vi "GainsToString.vi"(11 "Gains":T2) -> (3 "Strings":string[](array[string]))   [LabVIEW 2017]
uses:
  <vilib>/Analysis/Matrix/Datatypes/RealMatrix.ctl
  <vilib>/Analysis/Matrix/NI_Matrix.lvlib
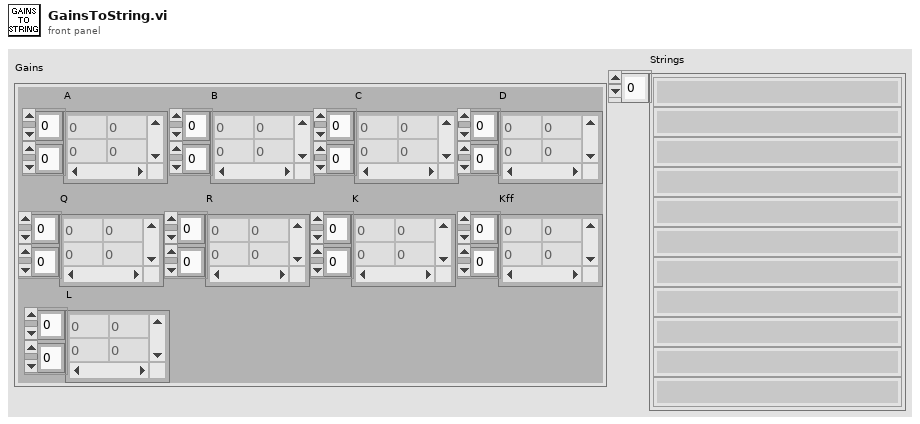
[diagram p1: front panel]
types:
  T1 = typedef "NI_Matrix.lvlib/RealMatrix.ctl" = dbl[][]
  T2 = cluster{"A":T1, "B":T1, "C":T1, "D":T1, "Q":T1, "R":T1, "K":T1, "Kff":T1, "L":T1}
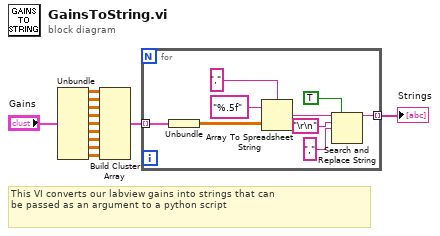
[diagram p0: block diagram]
diagram:
  # "This VI converts our labview gains into strings that can\nbe passed as an argument to a python script"
  n1 = Unbundle("Gains") -> ("A"=w1:T1, "B"=w11:T1, "C"=w10:T1, "D"=w9:T1, "Q"=w8:T1, "R"=w2:T1, "K"=w7:T1, "Kff"=w6:T1, "L"=w5:T1)
  n2 = Build Cluster Array(w1, w11, w10, w9, w8, w2, w7, w6, w5) -> (w4:cluster{"L":T1}[])
  n3 = for {
    tunnel: w4 -> [w14] mode=indexing
    tunnel: [w15] -> w3 mode=indexing
    n4 = Unbundle(w14) -> ("L"=w13:T1)
    n5 = Array To Spreadsheet String(delimiter (Tab)=",", array=w13, 3:"%.5f" ("format string")) -> (spreadsheet string=w16:string)
    n6 = Search and Replace String(replace all?=TRUE ("replace all? (F)"), input string=w16, search string="\r\n", replace string="," ("replace string (\"\")")) -> (result string=w15:string)  [unwired: 4 in, 3 out]
  }
  "Strings" <- w3
